vi "Handle Events.vi"(8 "error in (no error)":errorcluster, 11 "ControlEventHandler":refnum<class "ControlEventHandler.lvclass">) -> ()   [LabVIEW 2019, in "ActorEvents.lvlib" / "ControlEventHandler.lvclass"]
uses:
  <vilib>/gpm_packages/@cs/mva-viewable/Source/ActorEvents/EventHandler/ControlEventHandler/ControlEventHandler.lvclass
  C:/Program Files/National Instruments/LabVIEW 2019/vi.lib/gpm_packages/@cs/mva-viewable/Source/ActorEvents/IEventHandler/IEventHandler.lvclass
  <vilib>/gpm_packages/@cs/mva-viewable/Source/ActorEvents/EventHandler/ControlEventHandler/ControlEventHandler.lvclass/ControlEventHandler.ctl
  <vilib>/gpm_packages/@cs/mva-viewable/Source/ActorEvents/IEventHandler/IEventHandler.lvclass/IEventHandler.ctl
  <vilib>/ActorFramework/Message Enqueuer/Message Enqueuer.lvclass/Message Enqueuer.ctl
  <vilib>/gpm_packages/@cs/mva-viewable/Source/ActorEvents/IEventAggregator Messages/ControlMouseDownMsg/ControlMouseDownMsg.lvclass/ControlMouseDownMsg.ctl
  <vilib>/gpm_packages/@cs/mva-viewable/Source/ActorEvents/IEventAggregator Messages/EventDataMessage/EventDataMessage.lvclass/EventDataMessage.ctl
  <vilib>/gpm_packages/@cs/mva-viewable/Source/ActorEvents/IEventAggregator Messages/ControlKeyDownMsg/ControlKeyDownMsg.lvclass/ControlKeyDownMsg.ctl
  <vilib>/gpm_packages/@cs/mva-viewable/Source/ActorEvents/IEventAggregator Messages/ControlDragSourceUpdateMsg/ControlDragSourceUpdateMsg.lvclass/ControlDragSourceUpdateMsg.ctl
  <vilib>/event_ctls.llb/lveventtype.ctl
  <vilib>/gpm_packages/@cs/mva-viewable/Source/ActorEvents/IEventAggregator Messages/ControlMouseDownMsg/Accessors/Read Button.vi
  <vilib>/gpm_packages/@cs/mva-viewable/Source/ActorEvents/IEventAggregator Messages/ControlMouseDownMsg/Accessors/Read Mods.vi
  <vilib>/gpm_packages/@cs/mva-viewable/Source/ActorEvents/IEventAggregator Messages/ControlMouseDownMsg/Accessors/Read PlatMods.vi
  <vilib>/gpm_packages/@cs/mva-viewable/Source/ActorEvents/IEventAggregator Messages/EventDataMessage/Read Discarded.vi
  <vilib>/gpm_packages/@cs/mva-viewable/Source/ActorEvents/IEventAggregator Messages/ControlKeyDownMsg/Accessors/Read Char.vi
  <vilib>/gpm_packages/@cs/mva-viewable/Source/ActorEvents/IEventAggregator Messages/ControlKeyDownMsg/Accessors/Read VKey.vi
  <vilib>/gpm_packages/@cs/mva-viewable/Source/ActorEvents/IEventAggregator Messages/ControlKeyDownMsg/Accessors/Read Mods.vi
  <vilib>/gpm_packages/@cs/mva-viewable/Source/ActorEvents/IEventAggregator Messages/ControlKeyDownMsg/Accessors/Read PlatMods.vi
  <vilib>/gpm_packages/@cs/mva-viewable/Source/ActorEvents/IEventAggregator Messages/ControlKeyDownMsg/Accessors/Read FocusObj.vi
  <vilib>/gpm_packages/@cs/mva-viewable/Source/ActorEvents/IEventAggregator Messages/ControlDragSourceUpdateMsg/Accessors/Read Cursor.vi
  <vilib>/gpm_packages/@cs/mva-viewable/Source/ActorEvents/IEventHandler/Accessors/Read Timeout [ms].vi
  <vilib>/gpm_packages/@cs/mva-viewable/Source/ActorEvents/IEventHandler/Accessors/Read Event Filter.vi
  <vilib>/gpm_packages/@cs/mva-viewable/Source/ActorEvents/IEventHandler/Accessors/Read EventAggregator Enqueuer.vi
  <vilib>/gpm_packages/@cs/mva-viewable/Source/ActorEvents/IEventHandler/Accessors/Read Timeout Message.vi
  <vilib>/gpm_packages/@cs/mva-viewable/Source/ActorEvents/IEventHandler/Accessors/Read Timeout Message Priority.vi
  <vilib>/gpm_packages/@cs/mva-viewable/Source/ActorEvents/IEventAggregator Messages/ControlMouseDownMsg/ControlMouseDownMsg.lvclass
  C:/Program Files/National Instruments/LabVIEW 2019/vi.lib/gpm_packages/@cs/mva-viewable/Source/ActorEvents/IEventAggregator Messages/EventDataMessage/EventDataMessage.lvclass
  <vilib>/gpm_packages/@cs/mva-viewable/Source/ActorEvents/IEventAggregator Messages/ControlKeyDownMsg/ControlKeyDownMsg.lvclass
  <vilib>/gpm_packages/@cs/mva-viewable/Source/ActorEvents/IEventAggregator Messages/ControlDropMsg/ControlDropMsg.lvclass
  <vilib>/gpm_packages/@cs/mva-viewable/Source/ActorEvents/IEventAggregator Messages/ControlDragOverMsg/ControlDragOverMsg.lvclass
  <vilib>/gpm_packages/@cs/mva-viewable/Source/ActorEvents/IEventAggregator Messages/ControlDragSourceUpdateMsg/ControlDragSourceUpdateMsg.lvclass
  <vilib>/gpm_packages/@cs/mva-viewable/Source/ActorEvents/IEventAggregator Messages/ShortcutMenuActivationMsg/ShortcutMenuActivationMsg.lvclass
  <vilib>/gpm_packages/@cs/mva-viewable/Source/ActorEvents/IEventAggregator Messages/ShortcutMenuSelectionMsg/ShortcutMenuSelectionMsg.lvclass
  <vilib>/ActorFramework/Message Priority Queue/Priority Enqueue.vi
  <vilib>/gpm_packages/@cs/mva-viewable/Source/ActorEvents/IEventFilter/IEventFilter.lvclass
  <vilib>/ActorFramework/Message Enqueuer/Message Enqueuer.lvclass
  <vilib>/ActorFramework/Message/Message.lvclass
  <vilib>/gpm_packages/@cs/mva-viewable/Source/ActorEvents/IEventAggregator Messages/ValueChangeMsg/ValueChangeMsg.lvclass
  <vilib>/gpm_packages/@cs/mva-viewable/Source/ActorEvents/IEventAggregator Messages/ControlMouseUpMsg/ControlMouseUpMsg.lvclass
  <vilib>/gpm_packages/@cs/mva-viewable/Source/ActorEvents/IEventAggregator Messages/ControlMouseEnterMsg/ControlMouseEnterMsg.lvclass
  <vilib>/gpm_packages/@cs/mva-viewable/Source/ActorEvents/IEventAggregator Messages/ControlMouseLeaveMsg/ControlMouseLeaveMsg.lvclass
  <vilib>/gpm_packages/@cs/mva-viewable/Source/ActorEvents/IEventAggregator Messages/ControlKeyUpMsg/ControlKeyUpMsg.lvclass
  <vilib>/gpm_packages/@cs/mva-viewable/Source/ActorEvents/IEventAggregator Messages/ControlDragEndedMsg/ControlDragEndedMsg.lvclass
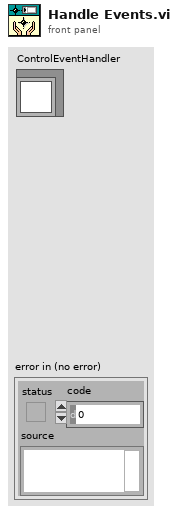
[diagram p1: front panel]
types:
  T1 = typedef "ActorEvents.lvlib/IEventFilter.lvclass/EventFilter Reference.ctl" = refnum<data-value>
  T2 = typedef "Actor Framework.lvlib/Message Enqueuer.lvclass/Message Priority.ctl" = enum16{"Low", "Normal", "High"}
  T3 = typedef "lveventtype.ctl" = enum32{"Null", "Timeout", "Annotation Menu Selection", "Annotation Menu Selection?", "App Instance Close", "App Instance Close?", "Autoscale Range Change", "Bookmark Info Change", "Cell Edit", "Cell Edit?", "Cursor Grab", "Cursor Grab?", "Cursor Menu Selection", "Cursor Menu Selection?", "Cursor Move", "Cursor Release", "Data Change", "Direction Change", "Display State Change", "Drag Ended", "Drag Enter", "Drag Leave", "Drag Over", "Drag Source Update", "Drag Starting", "Drag Starting?", "Drop", "Exec State Change", "Key Down", "Key Down?", "Key Repeat", "Key Repeat?", "Key Up", "Listbox Double Click", "Menu Activation?", "Menu Selection (App)", "Menu Selection? (App)", "Menu Selection (User)", "Mouse Down", "Mouse Down?", "Mouse Enter", "Mouse Leave", "Mouse Move", "Mouse Up", "Mouse Wheel", "NI Security User Change (App)", "Pane Size", "Panel Close", "Panel Close?", "Panel Resize", "Plot Attribute Change", "Scale Range Change", "Shortcut Menu Activation?", "Shortcut Menu Selection (App)", "Shortcut Menu Selection? (App)", "Shortcut Menu Selection (User)", "Tree Double Click", "Tree Drag", "Tree Drag?", "Tree Drop", "Tree Drop?", "Tree Item Close", "Tree Item Close?", "Tree Item Open", "Tree Item Open?", "User Event", "Value Change"}
  T4 = typedef "LVPoint32TypeDef.ctl" = cluster{"Horizontal":i32, "Vertical":i32}
  T5 = cluster{"Shift":bool, "Ctrl":bool, "Alt":bool, "Cmd":bool, "Opt":bool}
  T6 = typedef "eventvkey.ctl" = enum16{"ASCII", "Enter", "Return", "Shift", "Ctrl", "Alt", "Cmd", "Opt", "Caps", "NumLock", "Clear", "Break", "Up", "Down", "Left", "Right", "Insert", "Delete", "Home", "End", "PageUp", "PageDown", "Escape", "Help", "Pause", "ScrollLock", "F1", "F2", "F3", "F4", "F5", "F6", "F7", "F8", "F9", "F10", "F11", "F12", "F13", "F14", "F15", "F16", "F17", "F18", "F19", "F20", "F21", "F22", "F23", "F24", "Play", "VolumeUp", "VolumeDown", "Mute", "Two Byte Char"}
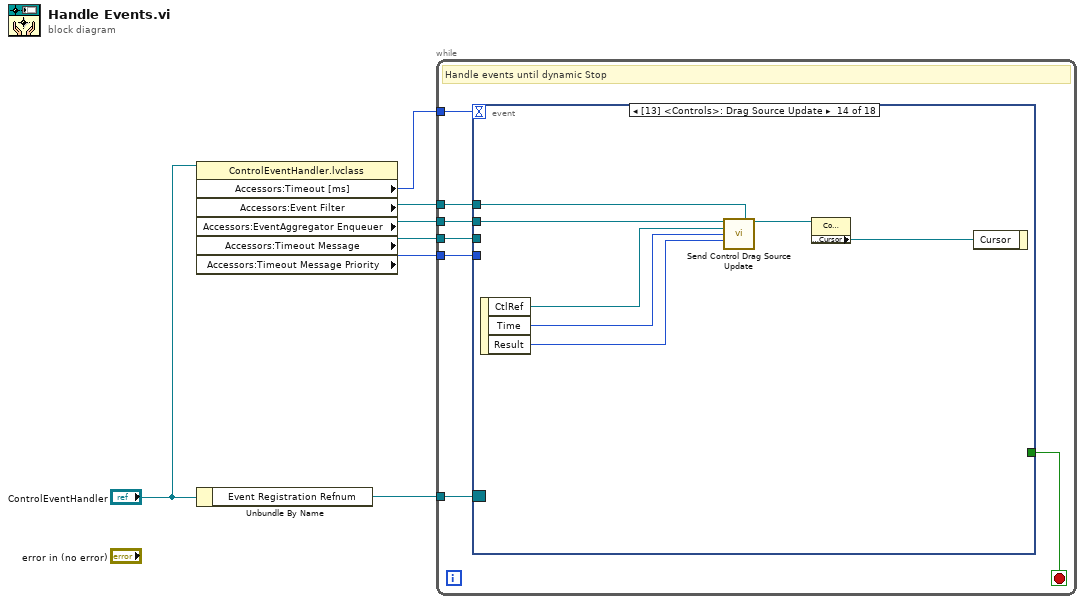
[diagram p0: block diagram]
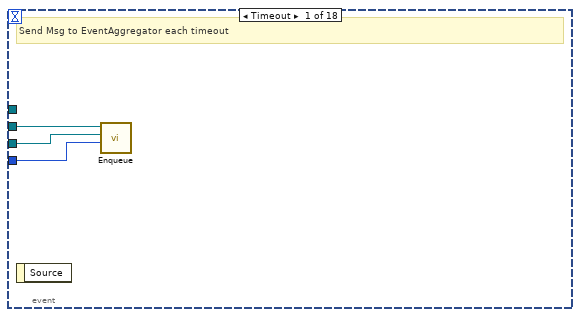
[diagram p2: hidden frame]
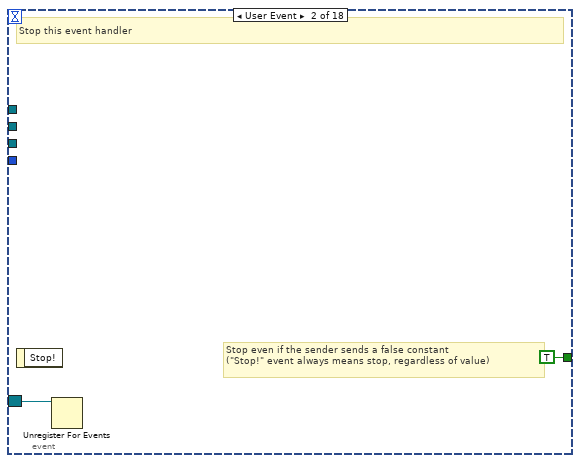
[diagram p3: hidden frame]
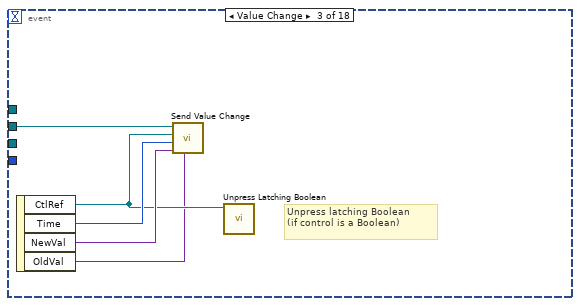
[diagram p4: hidden frame]
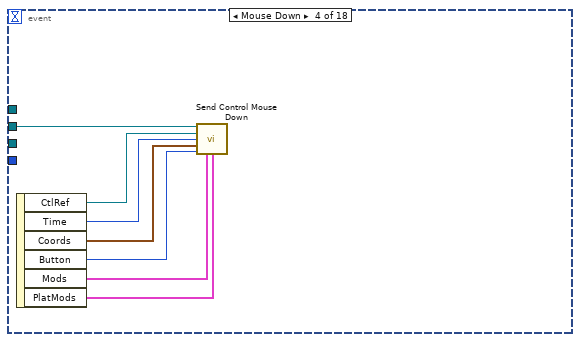
[diagram p5: hidden frame]
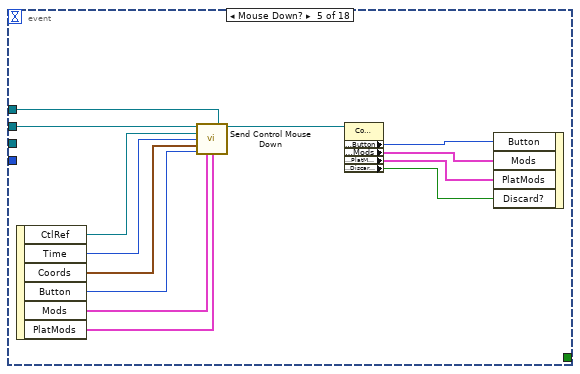
[diagram p6: hidden frame]
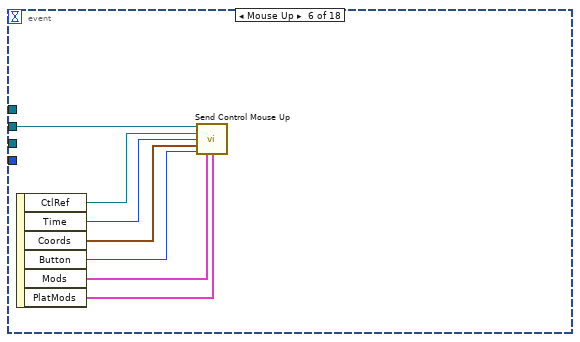
[diagram p7: hidden frame]
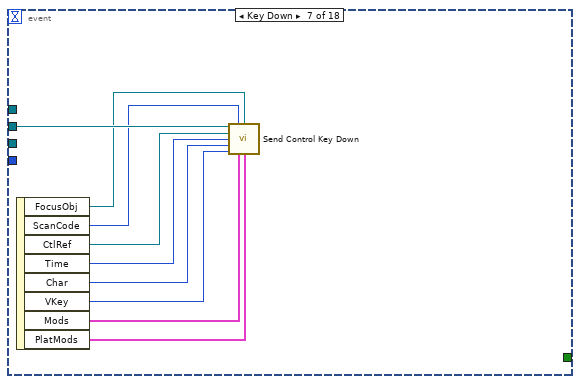
[diagram p8: hidden frame]
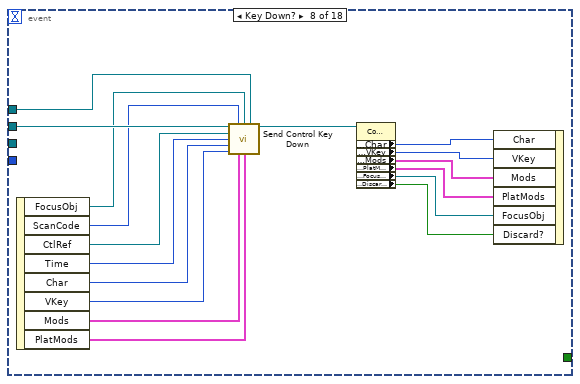
[diagram p9: hidden frame]
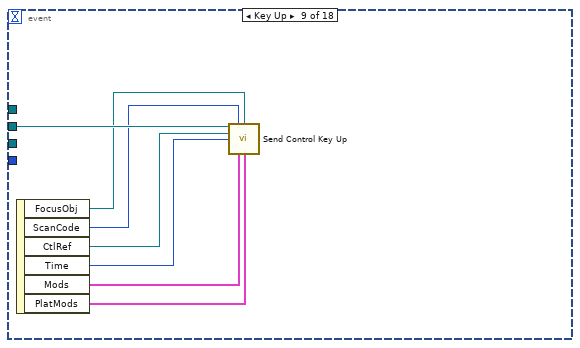
[diagram p10: hidden frame]
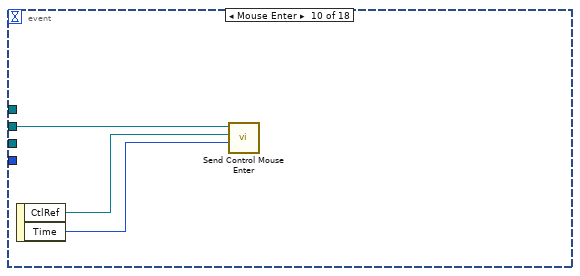
[diagram p11: hidden frame]
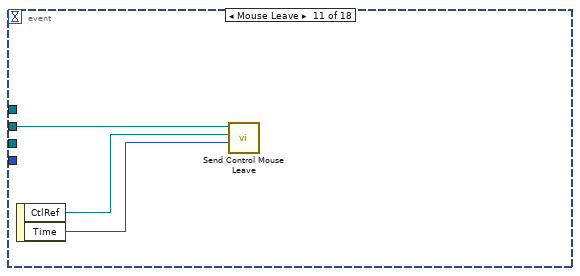
[diagram p12: hidden frame]
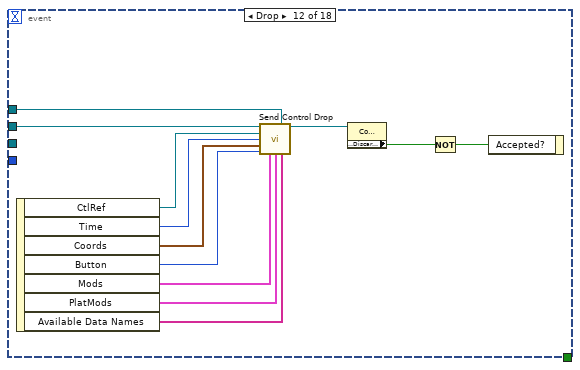
[diagram p13: hidden frame]
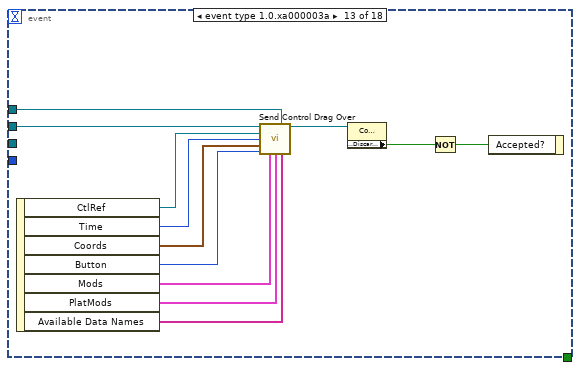
[diagram p14: hidden frame]
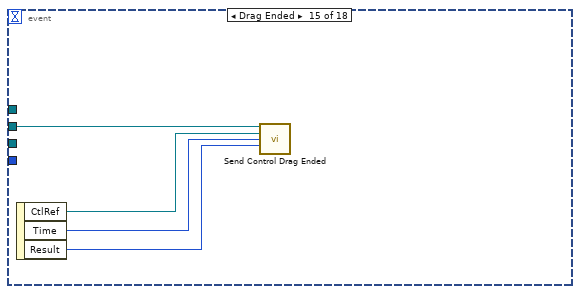
[diagram p15: hidden frame]
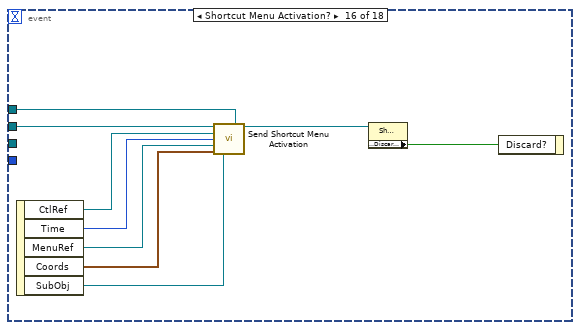
[diagram p16: hidden frame]
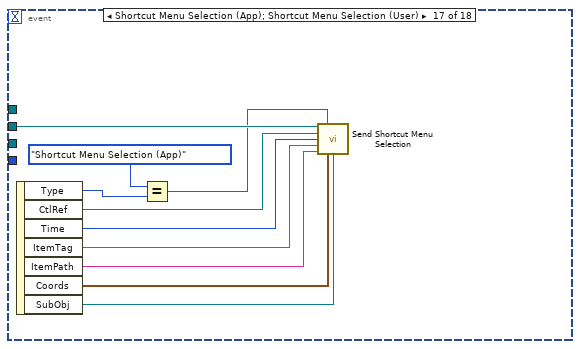
[diagram p17: hidden frame]
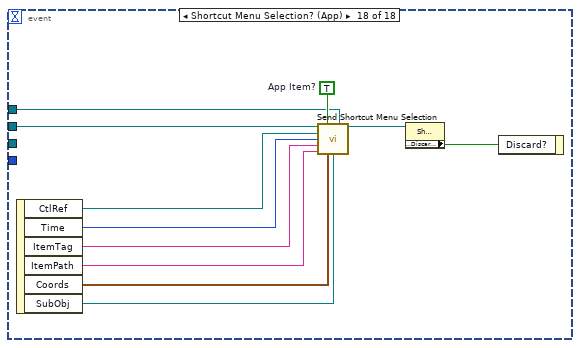
[diagram p18: hidden frame]
diagram:
  n1 = property class="ControlEventHandler.lvclass"(reference="ControlEventHandler") -> ("Accessors:Timeout [ms]"=w1:i32, "Accessors:Event Filter"=w2:T1, "Accessors:EventAggregator Enqueuer"=w5:refnum<class "Message Enqueuer.lvclass">, "Accessors:Timeout Message"=w4:refnum<class "Message.lvclass">, "Accessors:Timeout Message Priority"=w3:T2)  [unwired: 1 in, 2 out]
  n2 = Unbundle By Name("ControlEventHandler") -> ("Event Registration Refnum"=w7:refnum<event-registration>)
  n3 = while {
    tunnel: w7 -> [w14]
    tunnel: w5 -> [w13]
    tunnel: w4 -> [w12]
    tunnel: w3 -> [w11]
    tunnel: w2 -> [w9]
    tunnel: w1 -> [w8]
    stop <- w10 stop-if-true
    # "Handle events until dynamic Stop"
    n4 = event shown="[13] <Controls>: Drag Source Update" {
      selector: w14 -> [_ w19 _ _ _ _ _ _ _ _ _ _ _ _ _ _ _ _]
      dyn-events: _ -> [_ _ _ _ _ _ _ _ _ _ _ _ _ _ _ _ _ _]
      timeout: w8 -> [_ _ _ _ _ _ _ _ _ _ _ _ _ _ _ _ _ _]
      tunnel: w13 -> [w17 _ w24 w31 w44 w51 w60 w77 w84 w87 w90 w102 w114 w121 w125 w134 w144 w155]
      tunnel: w12 -> [w16 _ _ _ _ _ _ _ _ _ _ _ _ _ _ _ _ _]
      tunnel: w11 -> [w15 _ _ _ _ _ _ _ _ _ _ _ _ _ _ _ _ _]
      tunnel: [_ TRUE ("Stop!") _ _ _ _ _ _ _ _ _ _ _ _ _ _ _ _] -> w10
      tunnel: w9 -> [_ _ _ _ w32 _ _ w68 _ _ _ w94 w106 w118 _ w128 _ w145]
      event Timeout {
        # "Send Msg to EventAggregator each timeout"
        n5 = event-data() -> ()  [unwired: 1 in, 1 out]
        n6 = call <vilib>:"Enqueue.vi"("Message Priority (Normal)"=w15, "Message"=w16, "Message Enqueuer in"=w17) -> ()  [unwired: 7 in, 2 out]
      }
      event User Event {
        # "Stop even if the sender sends a false constant\n(\"Stop!\" event always means stop, regardless of value)"
        # "Stop this event handler"
        n7 = event-data() -> ()  [unwired: 1 in, 1 out]
        n8 = Unregister For Events(event registration refnum=w19) -> ()  [unwired: 1 in, 1 out]
      }
      event Value Change {
        # "Unpress latching Boolean\n(if control is a Boolean)"
        n9 = event-data() -> ("CtlRef"=w21:refnum<vi>, "Time"=w23:u32, "NewVal"=w22:variant, "OldVal"=w20:variant)  [unwired: 1 in]
        n10 = call <vilib>:"Send Value Change.vi"("Old Value"=w20, "New Value"=w22, "Time"=w23, "Ctl Refnum"=w21, "Message Enqueuer in"=w24) -> ()  [unwired: 6 in, 1 out]
        n11 = call <vilib>:"Unpress Latching Boolean.vi"("Ctl Refnum"=w21) -> ()  [unwired: 11 in]
      }
      event Mouse Down {
        n12 = event-data() -> ("CtlRef"=w30:refnum<vi>, "Time"=w29:u32, "Coords"=w28:T4, "Button"=w27:u16, "Mods"=w26:cluster{"Double Click":bool, "Menu Key":bool}, "PlatMods"=w25:T5)  [unwired: 1 in]
        n13 = call <vilib>:"Send Control Mouse Down.vi"("Message Enqueuer in"=w31, "Ctl Refnum"=w30, "Time"=w29, "Coords"=w28, "Button"=w27, "Mods"=w26, "PlatMods"=w25) -> ()  [unwired: 7 in, 2 out]
      }
      event Mouse Down? {
        n14 = event-data() -> ("CtlRef"=w43:refnum<vi>, "Time"=w42:u32, "Coords"=w41:T4, "Button"=w40:u16, "Mods"=w39:cluster{"Double Click":bool, "Menu Key":bool}, "PlatMods"=w38:T5)  [unwired: 1 in]
        n15 = call <vilib>:"Send Control Mouse Down.vi"("Message Enqueuer in"=w44, "EventFilter Reference"=w32, "Ctl Refnum"=w43, "Time"=w42, "Coords"=w41, "Button"=w40, "Mods"=w39, "PlatMods"=w38) -> ("Filtered EventDataMessage"=w37:refnum<class "ControlMouseDownMsg.lvclass">)  [unwired: 6 in, 1 out]
        n16 = property class="ControlMouseDownMsg.lvclass"(reference=w37) -> ("Accessors:Button"=w36:u16, "Accessors:Mods"=w35:cluster{"Double Click":bool, "Menu Key":bool}, "Accessors:PlatMods"=w34:T5, "Accessors:Discarded?"=w33:bool)  [unwired: 1 in, 2 out]
        n17 = event-data("Button"=w36, "Mods"=w35, "PlatMods"=w34, "Discard?"=w33) -> ()  [unwired: 1 in, 1 out]
      }
      event Mouse Up {
        n18 = event-data() -> ("CtlRef"=w50:refnum<vi>, "Time"=w49:u32, "Coords"=w48:T4, "Button"=w47:u16, "Mods"=w46:cluster{"Double Click":bool, "Menu Key":bool}, "PlatMods"=w45:T5)  [unwired: 1 in]
        n19 = call <vilib>:"Send Control Mouse Up.vi"("Message Enqueuer in"=w51, "Ctl Refnum"=w50, "Time"=w49, "Coords"=w48, "Button"=w47, "Mods"=w46, "PlatMods"=w45) -> ()  [unwired: 8 in, 1 out]
      }
      event Key Down {
        n20 = event-data() -> ("FocusObj"=w53:refnum<vi>, "ScanCode"=w52:i16, "CtlRef"=w59:refnum<vi>, "Time"=w58:u32, "Char"=w57:i16, "VKey"=w54:T6, "Mods"=w56:cluster{"Num Pad":bool, "Menu Key":bool}, "PlatMods"=w55:T5)  [unwired: 1 in]
        n21 = call <vilib>:"Send Control Key Down.vi"("Message Enqueuer in"=w60, "ScanCode"=w52, "FocusObj"=w53, "CtlRef"=w59, "Time"=w58, "Char"=w57, "VKey"=w54, "Mods"=w56, "PlatMods"=w55) -> ()  [unwired: 5 in, 2 out]
      }
      event Key Down? {
        n22 = event-data() -> ("FocusObj"=w70:refnum<vi>, "ScanCode"=w69:i16, "CtlRef"=w76:refnum<vi>, "Time"=w75:u32, "Char"=w74:i16, "VKey"=w71:T6, "Mods"=w73:cluster{"Num Pad":bool, "Menu Key":bool}, "PlatMods"=w72:T5)  [unwired: 1 in]
        n23 = call <vilib>:"Send Control Key Down.vi"("Message Enqueuer in"=w77, "ScanCode"=w69, "FocusObj"=w70, "EventFilter Reference"=w68, "CtlRef"=w76, "Time"=w75, "Char"=w74, "VKey"=w71, "Mods"=w73, "PlatMods"=w72) -> ("Filtered EventDataMessage"=w67:refnum<class "ControlKeyDownMsg.lvclass">)  [unwired: 4 in, 1 out]
        n24 = property class="ControlKeyDownMsg.lvclass"(reference=w67) -> ("Accessors:Char"=w66:i16, "Accessors:VKey"=w65:T6, "Accessors:Mods"=w64:cluster{"Double Click":bool, "Menu Key":bool}, "Accessors:PlatMods"=w63:T5, "Accessors:FocusObj"=w62:refnum<vi>, "Accessors:Discarded?"=w61:bool)  [unwired: 1 in, 2 out]
        n25 = event-data("Char"=w66, "VKey"=w65, "Mods"=w64, "PlatMods"=w63, "FocusObj"=w62, "Discard?"=w61) -> ()  [unwired: 1 in, 1 out]
      }
      event Key Up {
        n26 = event-data() -> ("FocusObj"=w79:refnum<vi>, "ScanCode"=w78:i16, "CtlRef"=w83:refnum<vi>, "Time"=w82:u32, "Mods"=w81:cluster{"Num Pad":bool, "Menu Key":bool}, "PlatMods"=w80:T5)  [unwired: 1 in]
        n27 = call <vilib>:"Send Control Key Up.vi"("Message Enqueuer in"=w84, "ScanCode"=w78, "FocusObj"=w79, "Ctl Refnum"=w83, "Time"=w82, "Mods"=w81, "PlatMods"=w80) -> ()  [unwired: 8 in, 1 out]
      }
      event Mouse Enter {
        n28 = event-data() -> ("CtlRef"=w86:refnum<vi>, "Time"=w85:u32)  [unwired: 1 in]
        n29 = call <vilib>:"Send Control Mouse Enter.vi"("Time"=w85, "Ctl Refnum"=w86, "Message Enqueuer in"=w87) -> ()  [unwired: 8 in, 1 out]
      }
      event Mouse Leave {
        n30 = event-data() -> ("CtlRef"=w89:refnum<vi>, "Time"=w88:u32)  [unwired: 1 in]
        n31 = call <vilib>:"Send Control Mouse Leave.vi"("Time"=w88, "Ctl Refnum"=w89, "Message Enqueuer in"=w90) -> ()  [unwired: 8 in, 1 out]
      }
      event Drop {
        n32 = event-data() -> ("CtlRef"=w101:refnum<vi>, "Time"=w100:u32, "Coords"=w99:T4, "Button"=w98:u16, "Mods"=w97:cluster{"Double Click":bool, "Menu Key":bool}, "PlatMods"=w96:T5, "Available Data Names"=w95:string[])  [unwired: 1 in]
        n33 = call <vilib>:"Send Control Drop.vi"("Message Enqueuer in"=w102, "EventFilter Reference"=w94, "CtlRef"=w101, "Time"=w100, "Coords"=w99, "Button"=w98, "Mods"=w97, "PlatMods"=w96, "Available Data Names"=w95) -> ("Filtered EventDataMessage"=w93:refnum<class "ControlDropMsg.lvclass">)  [unwired: 5 in, 1 out]
        n34 = property class="ControlDropMsg.lvclass"(reference=w93) -> ("Accessors:Discarded?"=w92:bool)  [unwired: 1 in, 2 out]
        n35 = Not(x=w92) -> (.not. x?=w91:bool)
        n36 = event-data("Accepted?"=w91) -> ()  [unwired: 1 in, 1 out]
      }
      event event type 1.0.xa000003a {
        n37 = event-data() -> ("CtlRef"=w113:refnum<vi>, "Time"=w112:u32, "Coords"=w111:T4, "Button"=w110:u16, "Mods"=w109:cluster{"Double Click":bool, "Menu Key":bool}, "PlatMods"=w108:T5, "Available Data Names"=w107:string[])  [unwired: 1 in]
        n38 = call <vilib>:"Send Control Drag Over.vi"("Message Enqueuer in"=w114, "EventFilter Reference"=w106, "CtlRef"=w113, "Time"=w112, "Coords"=w111, "Button"=w110, "Mods"=w109, "PlatMods"=w108, "Available Data Names"=w107) -> ("Filtered EventDataMessage"=w105:refnum<class "ControlDragOverMsg.lvclass">)  [unwired: 5 in, 1 out]
        n39 = property class="ControlDragOverMsg.lvclass"(reference=w105) -> ("Accessors:Discarded?"=w104:bool)  [unwired: 1 in, 2 out]
        n40 = Not(x=w104) -> (.not. x?=w103:bool)
        n41 = event-data("Accepted?"=w103) -> ()  [unwired: 1 in, 1 out]
      }
      event Drag Source Update {
        n42 = event-data() -> ("CtlRef"=w120:refnum<vi>, "Time"=w119:u32, "Result"=w115:enum16{"Drop Cancel", "Drop Move", "Drop Copy"})  [unwired: 1 in]
        n43 = call <vilib>:"Send Control Drag Source Update.vi"("Message Enqueuer in"=w121, "EventFilter Reference"=w118, "CtlRef"=w120, "Time"=w119, "Result"=w115) -> ("Filtered EventDataMessage"=w117:refnum<class "ControlDragSourceUpdateMsg.lvclass">)  [unwired: 9 in, 1 out]
        n44 = property class="ControlDragSourceUpdateMsg.lvcl"(reference=w117) -> ("Accessors:Cursor"=w116:refnum<k1>)  [unwired: 1 in, 2 out]
        n45 = event-data("Cursor"=w116) -> ()  [unwired: 1 in, 1 out]
      }
      event Drag Ended {
        n46 = event-data() -> ("CtlRef"=w124:refnum<vi>, "Time"=w123:u32, "Result"=w122:enum16{"Drop Cancel", "Drop Move", "Drop Copy"})  [unwired: 1 in]
        n47 = call <vilib>:"Send Control Drag Ended.vi"("Message Enqueuer in"=w125, "CtlRef"=w124, "Time"=w123, "Result"=w122) -> ()  [unwired: 10 in, 2 out]
      }
      event Shortcut Menu Activation? {
        n48 = event-data() -> ("CtlRef"=w133:refnum<vi>, "Time"=w132:u32, "MenuRef"=w131:refnum<k9>, "Coords"=w130:T4, "SubObj"=w129:refnum<vi>)  [unwired: 1 in]
        n49 = call <vilib>:"Send Shortcut Menu Activation.vi"("Message Enqueuer in"=w134, "EventFilter Reference"=w128, "CtlRef"=w133, "Time"=w132, "MenuRef"=w131, "Coords"=w130, "SubObj"=w129) -> ("Filtered EventDataMessage"=w127:refnum<class "ShortcutMenuActivationMsg.lvclass">)  [unwired: 7 in, 1 out]
        n50 = property class="ShortcutMenuActivationMsg.lvcla"(reference=w127) -> ("Accessors:Discarded?"=w126:bool)  [unwired: 1 in, 2 out]
        n51 = event-data("Discard?"=w126) -> ()  [unwired: 1 in, 1 out]
      }
      event Shortcut Menu Selection (App); Shortcut Menu Selection (User) {
        n52 = event-data() -> ("Type"=w137:T3, "CtlRef"=w143:refnum<vi>, "Time"=w142:u32, "ItemTag"=w141:string, "ItemPath"=w140:string, "Coords"=w138:T4, "SubObj"=w139:refnum<vi>)  [unwired: 1 in]
        n53 = Equal?(x=lveventtype."Shortcut Menu Selection (App)", y=w137) -> (x = y?=w135:bool)
        n54 = call <vilib>:"Send Shortcut Menu Selection.vi"("Message Enqueuer in"=w144, "App Item?"=w135, "CtlRef"=w143, "Time"=w142, "Item Tag"=w141, "Item Path"=w140, "Coords"=w138, "SubObj"=w139) -> ()  [unwired: 6 in, 2 out]
      }
      event Shortcut Menu Selection? (App) {
        w146 = TRUE  # App Item?
        n55 = event-data() -> ("CtlRef"=w154:refnum<vi>, "Time"=w153:u32, "ItemTag"=w152:string, "ItemPath"=w151:string, "Coords"=w149:T4, "SubObj"=w150:refnum<vi>)  [unwired: 1 in]
        n56 = call <vilib>:"Send Shortcut Menu Selection.vi"("Message Enqueuer in"=w155, "App Item?"=w146, "EventFilter Reference"=w145, "CtlRef"=w154, "Time"=w153, "Item Tag"=w152, "Item Path"=w151, "Coords"=w149, "SubObj"=w150) -> ("Filtered EventDataMessage"=w148:refnum<class "ShortcutMenuSelectionMsg.lvclass">)  [unwired: 5 in, 1 out]
        n57 = property class="ShortcutMenuSelectionMsg.lvclas"(reference=w148) -> ("Accessors:Discarded?"=w147:bool)  [unwired: 1 in, 2 out]
        n58 = event-data("Discard?"=w147) -> ()  [unwired: 1 in, 1 out]
      }
    }
  }
